vi "General PID Simulator with Alarm.vi"() -> ()   [LabVIEW 2023]
doc: "This example demonstrates how to simulate a general PID controller with alarms."
uses:
  <vilib>/addons/control/pid/pid.llb/PID (DBL).vi
  <vilib>/addons/control/pid/NI_PID_pid.lvlib
panel:
  out "Output":dbl(graph)
  out "Low Limit":bool
  out "High Limit":bool
  in  "Alarm":cluster{dbl, dbl}(slide)={24.183006535947708, 67.3202614379085} scale=0.0..100.0
  in  "SP:":dbl(slide)=54.966887417218544 min=0.0 max=0.0 scale=0.0..100.0
  out "MV:":dbl(slide)=100.0 scale=-100.0..100.0
  out "PV:":dbl(slide)=33.01408837398299 scale=0.0..100.0
  in  "PID gains":T1={"proportional gain (Kc)"=20.0, "integral time (Ti, min)"=0.008, "derivative time (Td, min)"=0.001} {"derivative time (Td, min)" format="%.3f"; "integral time (Ti, min)" format="%.3f"; "proportional gain (Kc)" format="%.3f"}
  in  "Stop":bool
  out "Monitor Chart":cluster{"initial PV":dbl, "SP:":dbl, dbl, dbl}(graph)
  # "Overview: This example demonstrates how to simulate a general PID controller with alarms.\nInstructions:\n1. Run the VI and observe the Process Variable (PV) following the Setpoint (SP) value.\n2. Move the setpoint above or below the High Limit (HL) or Low Limit (LL). Verify the controls flashing when limits are reached.\n3. Change the Alarm limits to a value above or below if you are changing HL or LL, respectively and verify that the controller stop flashing.\n3. Click Stop to stop the VI."
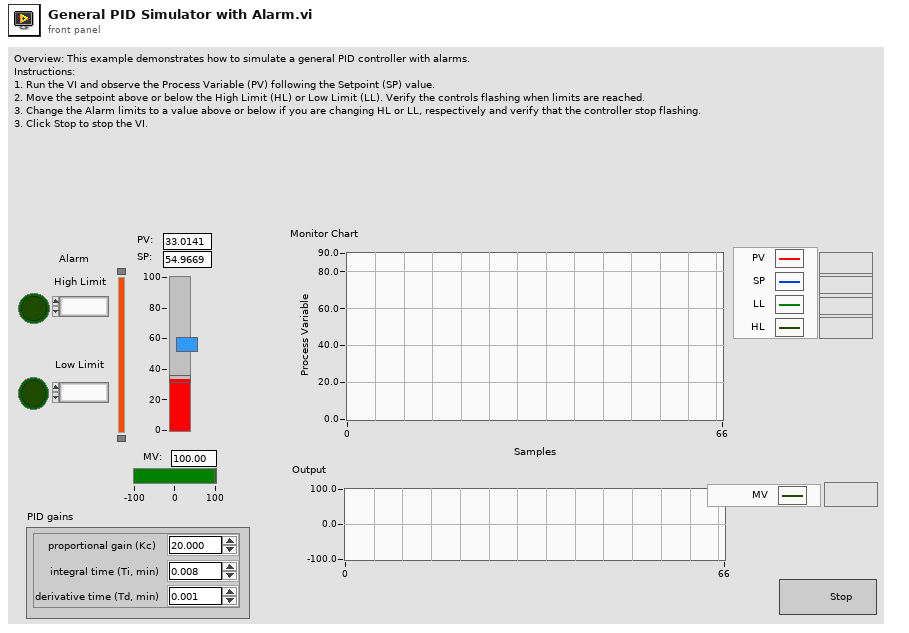
[diagram p1: front panel]
types:
  T1 = cluster{"proportional gain (Kc)":dbl, "integral time (Ti, min)":dbl, "derivative time (Td, min)":dbl}
  T2 = cluster{"static gain":dbl, "lag (min)":dbl, "dead cycles":dbl, "load %":dbl, "deadband":dbl, "noise level %":dbl, "initial PV":dbl, "initial PV 2":dbl}
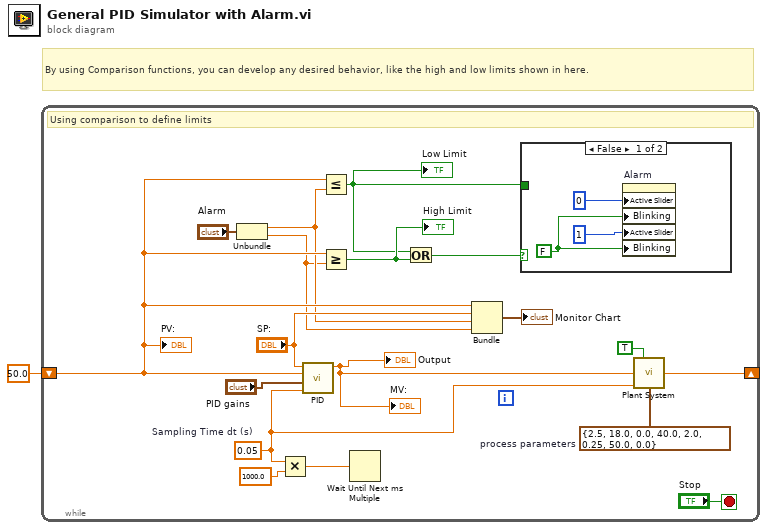
[diagram p0: block diagram]
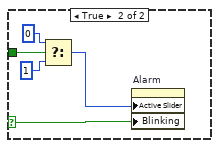
[diagram p2: hidden frame]
diagram:
  # "By using Comparison functions, you can develop any desired behavior, like the high and low limits shown in here."
  n1 = while {
    shift-left: 50.0 ("Plant Output") -> [w13]
    shift-right: [w17] -> _
    stop <- "Stop" stop-if-true
    w6 = T2 {"static gain"=2.5, "lag (min)"=18.0, "dead cycles"=0.0, "load %"=40.0, "deadband"=2.0, "noise level %"=0.25, "initial PV"=50.0, "initial PV 2"=0.0}  # process parameters
    w5 = 0.05  # Sampling Time dt (s)
    # "Using comparison to define limits"
    n2 = Unbundle("Alarm") -> (w11:dbl, w10:dbl)
    n3 = Multiply(x=w5, y=1000.0) -> (x*y=w2:dbl)
    n4 = call-poly <vilib>:"PID.vi"("dt (s)"=w5, "PID gains"="PID gains", "process variable"=w13, "setpoint"="SP:") -> ("output"=w3:dbl)  [unwired: 6 in, 1 out]
    "MV:" <- w3
    "Output" <- w3
    n5 = Less Or Equal?(x=w13, y=w11) -> (x <= y?=w7:bool)
    "Low Limit" <- w7
    n6 = Greater Or Equal?(x=w13, y=w10) -> (x >= y?=w9:bool)
    "High Limit" <- w9
    n7 = Wait Until Next ms Multiple(millisecond multiple=w2) -> ()  [unwired: 1 out]
    n8 = Or(x=w7, y=w9) -> (x .or. y?=w8:bool)
    n9 = Bundle("Plant Output"=w13, "SP:"="SP:", w11, w10) -> (→"Monitor Chart":cluster{"Plant Output":dbl, "SP:":dbl, dbl, dbl})  [unwired: 1 in]
    n10 = case shown="False" w8 {
      selector: w8 -> [_ w27]
      tunnel: w7 -> [_ w23]
      frame False {
        w21 = FALSE ("Blinking")
        n11 = property on="Alarm" class="Slide (strict)"("Active Slider"=0, "Blinking"=w21, "Active Slider"=1, "Blinking"=w21) -> ()  [unwired: 2 in, 2 out]
      }
      frame True {
        n12 = Select(t=0 ("Active Slider"), s=w23, f=1 ("Active Slider")) -> (s? t:f=w26:i32)
        n13 = property on="Alarm" class="Slide (strict)"("Active Slider"=w26, "Blinking"=w27) -> ()  [unwired: 2 in, 2 out]
      }
    }
    n14 = call "Plant System.vi"("Integrator ?"=TRUE, "Plant Input"=w3, "dt (s)"=w5, "process parameters"=w6) -> ("Plant Output"=w17:dbl)  [unwired: 11 in]
    "PV:" <- w13
  }
